vi "runTask.vi"(7 "SubPanel Ref":refnum<vi>, 8 "error in (no error)":errorcluster, 10 "Parameter":T1, 11 "Taskname":string) -> (0 "error out":errorcluster, 3 "Task Ref":refnum<vi>)   [LabVIEW 2015, in "pdbm_task_route.lvlib"]
uses:
  pdbm_task_route.lvlib
  UsrDefine/TaskFeedbackCmd.ctl
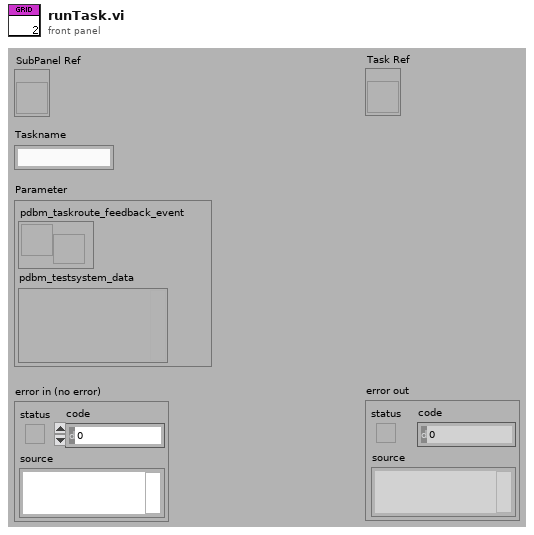
[diagram p1: front panel]
types:
  T1 = cluster{"pdbm_taskroute_feedback_event":refnum<user-event>, "pdbm_testsystem_data":variant}
  T2 = cluster{"pdbm_taskroute_feedback_event":refnum<user-event>, "pdbm_task_reqst_event":refnum<user-event>, "pdbm_testsystem_data":variant}
  T3 = enum32{"Bad", "Idle", "Run top level", "Running"}
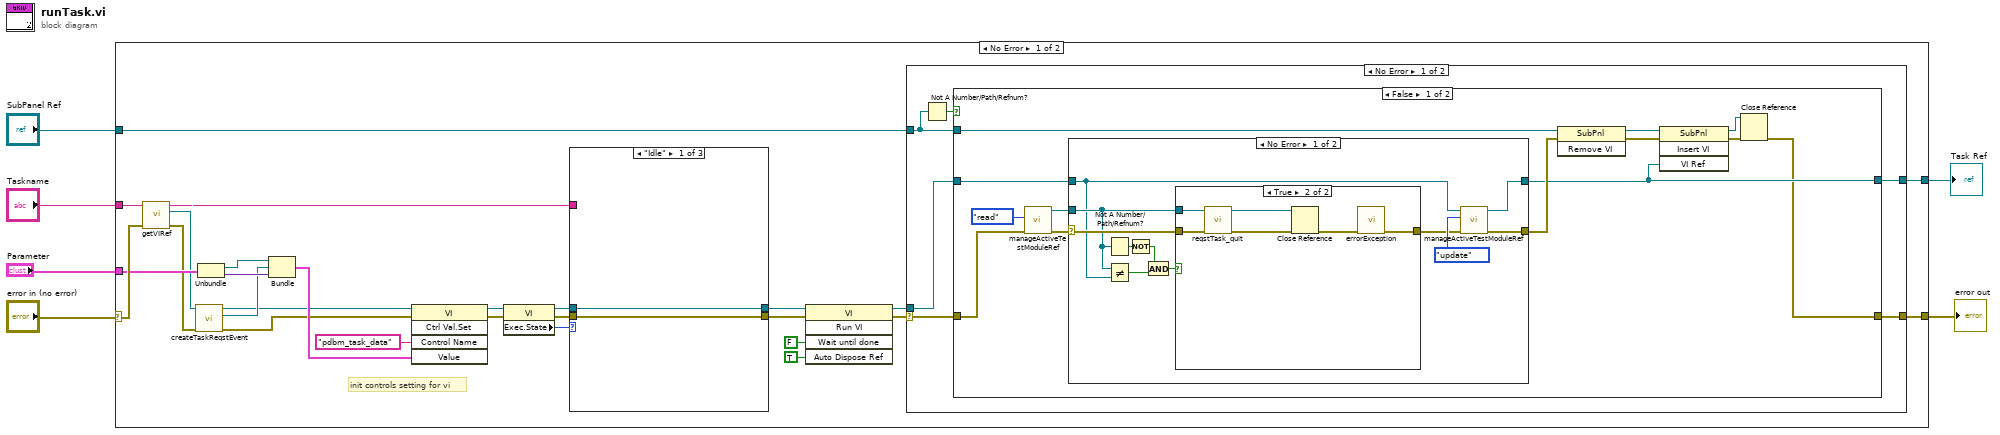
[diagram p0: block diagram]
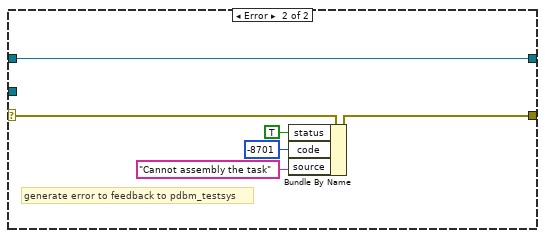
[diagram p3: hidden frame]
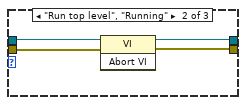
[diagram p6: hidden frame]
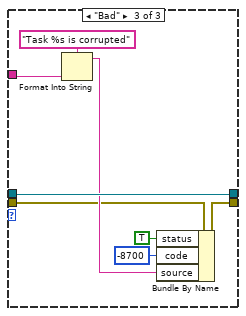
[diagram p7: hidden frame]
diagram:
  n1 = case shown="No Error" "error in (no error)" {
    selector: "error in (no error)" -> [w32 w95]
    tunnel: "Taskname" -> [w33 _]
    tunnel: "SubPanel Ref" -> [w27 _]
    tunnel: [w26 w95] -> w2
    tunnel: "Parameter" -> [w17 _]
    tunnel: [w25 _] -> w1
    frame No Error {
      # "init controls setting for vi"
      n2 = call "getVIRef.vi"("error in (no error)"=w32, "TaskName"=w33) -> ("error out"=w16:errorcluster, "Task Ref"=w15:refnum<vi>, "TaskName out"=w28:string)  [unwired: 7 in]
      n3 = call "createTaskReqstEvent.vi"("error in (no error)"=w16, "TaskRef"=w15) -> ("error IO"=w18:errorcluster, "pdbm_task_reqst_event"=w20:refnum<user-event>, "TaskRef out"=w19:refnum<vi>)  [unwired: 7 in]
      n4 = Unbundle(w17) -> ("pdbm_taskroute_feedback_event"=w23:refnum<user-event>, "pdbm_testsystem_data"=w22:variant)
      n5 = Bundle("pdbm_taskroute_feedback_event"=w23, "pdbm_task_reqst_event"=w20, "pdbm_testsystem_data"=w22) -> (w21:T2)  [unwired: 1 in]
      n6 = invoke class="VI" method="Ctrl Val.Set"(reference=w19, error in=w18, "Control Name"="pdbm_task_data", "Value"=w21) -> (reference out=w14:refnum<vi>, error out=w13:errorcluster)  [unwired: 1 in, 3 out]
      n7 = property class="VI"(reference=w14, error in=w13) -> (reference out=w30:refnum<vi>, error out=w29:errorcluster, "Exec.State"=w31:T3)
      n8 = case shown="\"Idle\"" w31 {
        tunnel: w30 -> [w82 w86 w91]
        tunnel: w29 -> [w81 w85 w87]
        tunnel: [w82 w84 w91] -> w10
        tunnel: [w81 w83 w94] -> w9
        tunnel: w28 -> [_ _ w90]
        frame "Idle" {
        }
        frame "Run top level", "Running" {
          n9 = invoke class="VI" method="Abort VI"(reference=w86, error in=w85) -> (reference out=w84:refnum<vi>, error out=w83:errorcluster)  [unwired: 1 in, 1 out]
        }
        frame "Bad" {
          n10 = Format Into String(format string="Task %s is corrupted" ("source"), w90) -> (resulting string=w88:string)  [unwired: 2 in, 1 out]
          n11 = Bundle By Name(cluster=w87, "status"=TRUE, "code"=-8700, "source"=w88) -> (w94:errorcluster)
        }
      }
      n12 = invoke class="VI" method="Run VI"(reference=w10, error in=w9, "Wait until done"=FALSE ("Wait Until Done"), "Auto Dispose Ref"=TRUE ("Auto Dispose Reference")) -> (reference out=w8:refnum<vi>, error out=w7:errorcluster)  [unwired: 1 in, 3 out]
      n13 = case shown="No Error" w7 {
        selector: w7 -> [w34 w80]
        tunnel: w8 -> [w35 w79]
        tunnel: w27 -> [w39 _]
        tunnel: [w37 w80] -> w26
        tunnel: [w36 w79] -> w25
        frame No Error {
          n14 = Not A Number/Path/Refnum?(number/path/refnum=w39) -> (NaN/Path/Refnum?=w38:bool)
          n15 = case shown="False" w38 {
            tunnel: w35 -> [w48 w77]
            tunnel: w34 -> [w50 w78]
            tunnel: w39 -> [w42 _]
            tunnel: [w40 w78] -> w37
            tunnel: [w41 w77] -> w36
            frame False {
              n16 = call "manageActiveTestModuleRef.vi"("error in (no error)"=w50, "operation"=enum16{"read", "update"}."read") -> ("error out"=w49:errorcluster, "ActiveTestModule Ref"=w51:refnum<vi>)  [unwired: 8 in]
              n17 = case shown="No Error" w49 {
                selector: w49 -> [w62 w73]
                tunnel: w51 -> [w58 _]
                tunnel: [w60 w72] -> w43
                tunnel: w48 -> [w57 w71]
                tunnel: [w59 w71] -> w41
                frame No Error {
                  n18 = Not A Number/Path/Refnum?(number/path/refnum=w58) -> (NaN/Path/Refnum?=w55:bool)
                  n19 = Not Equal?(x=w58, y=w57) -> (x != y?=w56:bool)
                  n20 = Not(x=w55) -> (.not. x?=w53:bool)
                  n21 = And(x=w53, y=w56) -> (x .and. y?=w54:bool)
                  n22 = case shown="True" w54 {
                    tunnel: w58 -> [_ w70]
                    tunnel: w62 -> [w64 w69]
                    tunnel: [w64 w65] -> w61
                    frame False {
                    }
                    frame True {
                      n23 = call "reqstTask_quit.vi"("error in (no error)"=w69, "TaskRef in"=w70) -> ("error IO"=w67:errorcluster, "TaskRef out"=w68:refnum<vi>)  [unwired: 8 in]
                      n24 = Close Reference(reference=w68, error in (no error)=w67) -> (error out=w66:errorcluster)
                      n25 = call "errorException.vi"("error in (no error)"=w66) -> ("error IO"=w65:errorcluster)  [unwired: 10 in]
                    }
                  }
                  n26 = call "manageActiveTestModuleRef.vi"("error in (no error)"=w61, "operation"=enum16{"read", "update"}."update", "New TestModule Ref"=w57) -> ("error out"=w60:errorcluster, "ActiveTestModule Ref"=w59:refnum<vi>)  [unwired: 7 in]
                }
                frame Error {
                  # "generate error to feedback to pdbm_testsys"
                  n27 = Bundle By Name(cluster=w73, "status"=TRUE, "code"=-8701, "source"="Cannot assembly the task") -> (w72:errorcluster)
                }
              }
              n28 = invoke class="SubPnl" method="Remove VI"(reference=w42, error in=w43) -> (reference out=w47:refnum<vi>, error out=w44:errorcluster)  [unwired: 1 in, 1 out]
              n29 = invoke class="SubPnl" method="Insert VI"(reference=w47, error in=w44, "VI Ref"=w41) -> (reference out=w45:refnum<vi>, error out=w46:errorcluster)  [unwired: 1 in, 2 out]
              n30 = Close Reference(reference=w45, error in (no error)=w46) -> (error out=w40:errorcluster)
            }
            frame True {
            }
          }
        }
        frame Error {
        }
      }
    }
    frame Error {
    }
  }
  "error out" <- w2
  "Task Ref" <- w1
